vi "Cube Drop.vi"   [LabVIEW 2020, in "VolatusSeq.lvlib"]
uses:
  VolatusSeq.lvlib
  VolatusSeqConfig/VolatusSeqConfig.lvlib
  OutOfRange Condition/OutOfRange Condition.lvclass
  LowLimit Condition/LowLimit Condition.lvclass
  HighLimit Condition/HighLimit Condition.lvclass
  Time Condition/Time Condition.lvclass
  State Transition/State Transition.lvclass
  SequencingHttpCtrlr/SequencingHttpCtrlr.lvclass
  Sequencing/Sequencing.lvclass
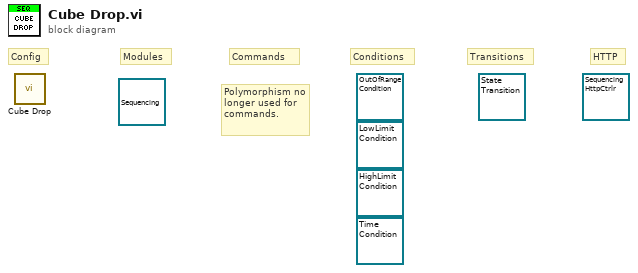
[diagram p0: block diagram]
diagram:
  (unwired) refnum<class "Sequencing.lvclass"> refnum ("VolatusSeq.lvlib:Sequencing.lvclass")
  (unwired) refnum<class "SequencingHttpCtrlr.lvclass"> refnum ("VolatusSeq.lvlib:SequencingHttpCtrlr.lvclass")
  (unwired) refnum<class "State Transition.lvclass"> refnum ("VolatusSeq.lvlib:State Transition.lvclass")
  (unwired) refnum<class "Time Condition.lvclass"> refnum ("VolatusSeq.lvlib:Time Condition.lvclass")
  (unwired) refnum<class "HighLimit Condition.lvclass"> refnum ("VolatusSeq.lvlib:HighLimit Condition.lvclass")
  (unwired) refnum<class "LowLimit Condition.lvclass"> refnum ("VolatusSeq.lvlib:LowLimit Condition.lvclass")
  (unwired) refnum<class "OutOfRange Condition.lvclass"> refnum ("VolatusSeq.lvlib:OutOfRange Condition.lvclass")
  # "Polymorphism no longer used for commands."
  # "HTTP"
  # "Transitions"
  # "Conditions"
  # "Commands"
  # "Modules"
  # "Config"
  n1 = call "Cube Drop.vi"() -> ()  [unwired: 12 in]
